vi "Sensor switch button (subVI).vi"(1 "Com found ?":bool, 2 "Input cluster":T1, 3 "Boolean in":refnum<vi>, 4 "First call?":bool) -> (0 "Output cluster 2":T1)   [LabVIEW 2016]
uses:
  Visa com cluster def (subVI).ctl
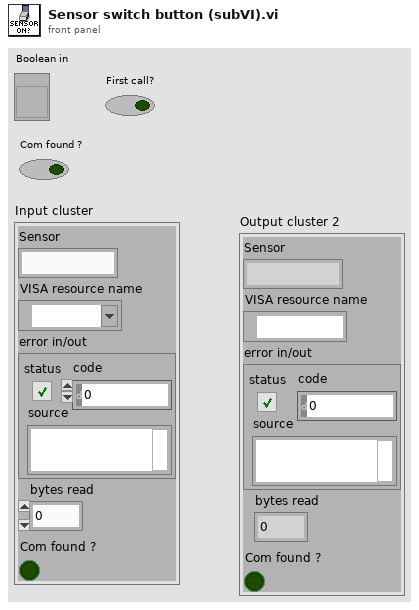
[diagram p1: front panel]
types:
  T1 = typedef "Visa com cluster def (subVI).ctl" = cluster{"Sensor":string, "VISA resource name":refnum<visa-resource-name>, "error in/out":errorcluster, "bytes read":u32, "Com found ?":bool}
  T2 = enum8{"Enabled", "Disabled", "Disabled and Grayed Out"}
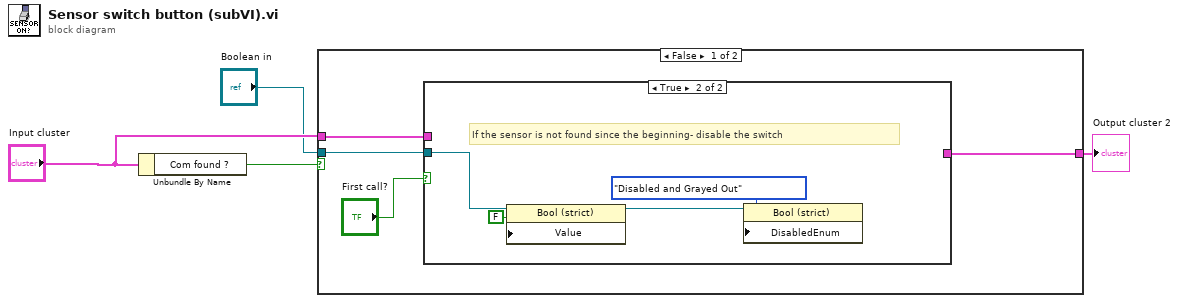
[diagram p0: block diagram]
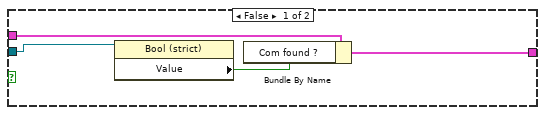
[diagram p2: hidden frame]
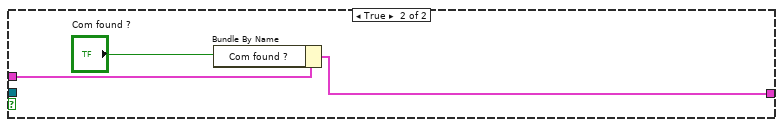
[diagram p3: hidden frame]
diagram:
  n1 = Unbundle By Name("Input cluster") -> ("Com found ?"=w3:bool)
  n2 = case shown="False" w3 {
    tunnel: "Input cluster" -> [w8 w18]
    tunnel: [w7 w17] -> w1
    tunnel: "Boolean in" -> [w6 _]
    frame False {
      n3 = case shown="True" "First call?" {
        tunnel: w8 -> [w11 _]
        tunnel: [w10 _] -> w7
        tunnel: w6 -> [w9 w14]
        frame False {
          n4 = property class="Bool (strict)"(reference=w9) -> ("Value"=w12:bool)  [unwired: 1 in, 2 out]
          n5 = Bundle By Name(cluster=w11, "Com found ?"=w12) -> (w10:T1)
        }
        frame True {
          # "If the sensor is not found since the beginning- disable the switch"
          n6 = property class="Bool (strict)"(reference=w14, "Value"=FALSE ("Com found ?")) -> (reference out=w13:refnum<vi>)  [unwired: 1 in, 1 out]
          n7 = property on="Property Node" class="Bool (strict)"(reference=w13, "DisabledEnum"=T2."Disabled and Grayed Out" ("Disabled")) -> ()  [unwired: 1 in, 2 out]
        }
      }
    }
    frame True {
      n8 = Bundle By Name(cluster=w18, "Com found ?"="Com found ?") -> (w17:T1)
    }
  }
  "Output cluster 2" <- w1
